vi "Configure Range.vi"(8 "error in (no error)":errorcluster, 9 "Current Range (Auto)":u16(ring) items=["Auto", "0.1Apk", "0.4Apk", "1.6Apk", "6.25Apk", "25Apk", "100Apk"], 10 "Voltage Range (Auto)":u16(ring) items=["Auto", "10Vpk", "46Vpk", "215Vpk", "900Vpk"], 11 "VISA resource name":refnum<visa-resource-name>) -> (0 "error out":errorcluster, 3 "VISA resource name out":refnum<visa-resource-name>)   [LabVIEW 2015, in "Voltech PM1000+.lvlib"]
doc: "Configures the ranges for both voltage and current. It also indicates the voltage and current range settings.\n\nFor most measurements, auto-ranging is the best choice. Choosing a fixed range\nmay be useful if the voltage or current is changing continuously or has large\npeaks which make the analyzer spend excessive time changing range."
uses:
  <instrlib>/Voltech PM1000+/Voltech PM1000+.lvlib
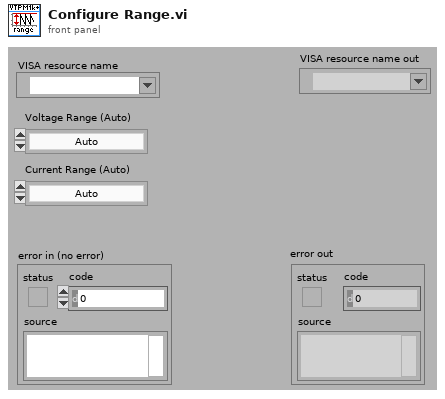
[diagram p1: front panel]
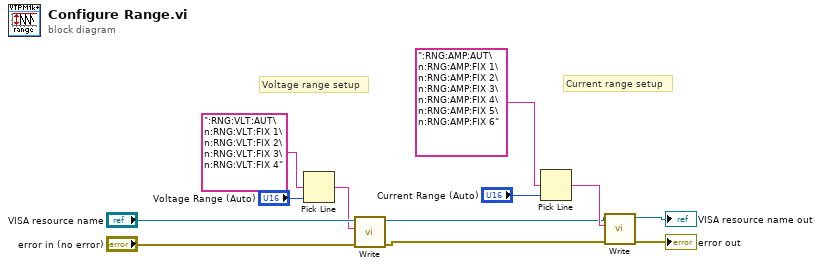
[diagram p0: block diagram]
diagram:
  # "Current range setup"
  # "Voltage range setup"
  n1 = Pick Line(multi-line string=":RNG:VLT:AUT\n:RNG:VLT:FIX 1\n:RNG:VLT:FIX 2\n:RNG:VLT:FIX 3\n:RNG:VLT:FIX 4", line index="Voltage Range (Auto)") -> (output string=w6:string)  [unwired: 1 in]
  n2 = call <instrlib>:"Write.vi"("error in (no error)"="error in (no error)", "Write Buffer"=w6, "VISA resource name"="VISA resource name") -> ("error out"=w3:errorcluster, "VISA resource name out"=w4:refnum<visa-resource-name>)  [unwired: 7 in]
  n3 = Pick Line(multi-line string=":RNG:AMP:AUT\n:RNG:AMP:FIX 1\n:RNG:AMP:FIX 2\n:RNG:AMP:FIX 3\n:RNG:AMP:FIX 4\n:RNG:AMP:FIX 5\n:RNG:AMP:FIX 6", line index="Current Range (Auto)") -> (output string=w5:string)  [unwired: 1 in]
  n4 = call <instrlib>:"Write.vi"("error in (no error)"=w3, "Write Buffer"=w5, "VISA resource name"=w4) -> ("error out"=→"error out":errorcluster, "VISA resource name out"=→"VISA resource name out":refnum<visa-resource-name>)  [unwired: 7 in]
